vi "Send MC Telemetry.vi"   [LabVIEW 2014]
uses:
  MC Telemetry.ctl
  MC Temp 1.ctl
  MC Temp 2.ctl
  MC Temp 3.ctl
  MC Current.ctl
  MC Voltage.ctl
  MC State.ctl
  Inverter States.ctl
  Inverter Run Modes.ctl
  VSM States.ctl
  MC Torque.ctl
  MC Faults.ctl
  MC Post Faults.ctl
  MC Run Faults.ctl
  MC Position.ctl
  Global Data.vi
types:
  T1 = typedef "MC Telemetry.ctl" = cluster{"MC Temp 1":T2, "MC Temp 2":T3, "MC Temp 3":T4, "MC Current":T5, "MC Voltage":T6, "MC State":T7, "MC Torque":T11, "MC Faults":T12, "MC Position":T15}
  T2 = typedef "MC Temp 1.ctl" = cluster{"IGBT A (C)":dbl, "IGBT B (C)":dbl, "IGBT C (C)":dbl, "Gate Driver (C)":dbl}
  T3 = typedef "MC Temp 2.ctl" = cluster{"Control Board (C)":dbl, "RTD #1":dbl, "RTD #2":dbl, "RTD #3":dbl}
  T4 = typedef "MC Temp 3.ctl" = cluster{"RTD #4":dbl, "RTD #5":dbl, "Motor (C)":dbl, "T-Shudder":dbl}
  T5 = typedef "MC Current.ctl" = cluster{"I-Phase A":dbl, "I-Phase B":dbl, "I-Phase C":dbl, "I-Battery":dbl}
  T6 = typedef "MC Voltage.ctl" = cluster{"V-Phase AB":dbl, "V-Phase BC":dbl, "V-Output":dbl, "V-Battery":dbl}
  T7 = typedef "MC State.ctl" = cluster{"Inverter":T8, "Inv. Run Mode":T9, "Inv. Command":enum16{"CAN Mode", "VSM Mode"}, "Inv. Enable":enum16{"Inverter Disabled", "Inverter Enabled"}, "Inv. Enable Lock":enum16{"Inverter Locked", "Inverter Unlocked"}, "Direction":enum16{"Forward", "Reverse/Stopped"}, "VSM States":T10, "Relay 1":bool, "Relay 2":bool, "Relay 3":bool, "Relay 4":bool}
  T8 = typedef "Inverter States.ctl" = enum16{"Power On", "Stop", "Open Loop", "Closed Loop", "Wait", "Internal", "Idle Run", "Idle Stop", ""}
  T9 = typedef "Inverter Run Modes.ctl" = enum16{"Torque Mode", "Speed Mode"}
  T10 = typedef "VSM States.ctl" = enum16{"VSM Start", "Pre-Charge Init", "Pre-Charge Active", "Pre-Charge Complete", "VSM Wait", "VSM Ready", "Motor Running", "Blink Fault Code", "Shutdown in Process", "Recycle Power"}
  T11 = typedef "MC Torque.ctl" = cluster{"T-Requested (Telem)":dbl, "T-Feedback":dbl}
  T12 = typedef "MC Faults.ctl" = cluster{"POST":T13, "RUN":T14}
  T13 = typedef "MC Post Faults.ctl" = enum32{"None"}
  T14 = typedef "MC Run Faults.ctl" = enum32{"None"}
  T15 = typedef "MC Position.ctl" = cluster{"Motor Angle":dbl, "Motor Speed":dbl, "Electrical Output Freq.":dbl, "Delta Resolver Filt.":dbl}
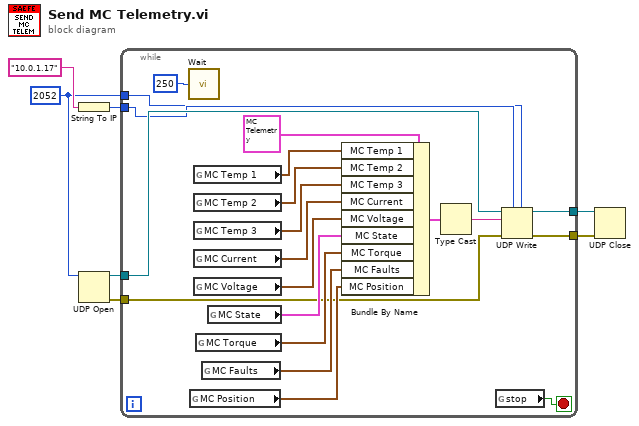
[diagram p0: block diagram]
diagram:
  w2 = u16 2052 ("port")
  n1 = String To IP(1:"10.0.1.17" ("name")) -> (0:w1:u32)
  n2 = UDP Open(11:w2) -> (port=w6:refnum<k16>, 0:w5:errorcluster)  [unwired: 4 in, 1 out]
  n3 = while {
    tunnel: w6 -> [w15]
    tunnel: w5 -> [w14]
    tunnel: [w11] -> w4
    tunnel: [w10] -> w3
    tunnel: w1 -> [w9]
    tunnel: w2 -> [w8]
    stop <- w26 stop-if-true
    n4 = call "Wait"("Count(mSec)"=u32 250) -> ()  [unwired: 1 out]
    n5 = global read "Global Data.vi" "MC Position"() -> (w16:T15)
    n6 = global read "Global Data.vi" "MC Temp 1"() -> (w24:T2)
    n7 = global read "Global Data.vi" "MC Temp 2"() -> (w23:T3)
    n8 = global read "Global Data.vi" "MC Temp 3"() -> (w22:T4)
    n9 = global read "Global Data.vi" "MC Current"() -> (w21:T5)
    n10 = global read "Global Data.vi" "MC Voltage"() -> (w20:T6)
    n11 = global read "Global Data.vi" "MC Torque"() -> (w18:T11)
    n12 = global read "Global Data.vi" "MC Faults"() -> (w17:T12)
    n13 = global read "Global Data.vi" "MC State"() -> (w19:T7)
    n14 = Bundle By Name(cluster=T1 {"MC Temp 1"={"IGBT A (C)"=0.0, "IGBT B (C)"=0.0, "IGBT C (C)"=0.0, "Gate Driver (C)"=0.0}, "MC Temp 2"={"Control Board (C)"=0.0, "RTD #1"=0.0, "RTD #2"=0.0, "RTD #3"=0.0}, "MC Temp 3"={"RTD #4"=0.0, "RTD #5"=0.0, "Motor (C)"=0.0, "T-Shudder"=0.0}, "MC Current"={"I-Phase A"=0.0, "I-Phase B"=0.0, "I-Phase C"=0.0, "I-Battery"=0.0}, "MC Voltage"={"V-Phase AB"=0.0, "V-Phase BC"=0.0, "V-Output"=0.0, "V-Battery"=0.0}, "MC State"={"Inverter"=enum."Power On", "Inv. Run Mode"=enum."Torque Mode", "Inv. Command"=enum."CAN Mode", "Inv. Enable"=enum."Inverter Disabled", "Inv. Enable Lock"=enum."Inverter Locked", "Direction"=enum."Forward", "VSM States"=enum."VSM Start", "Relay 1"=FALSE, "Relay 2"=FALSE, "Relay 3"=FALSE, "Relay 4"=FALSE}, "MC Torque"={"T-Requested (Telem)"=0.0, "T-Feedback"=0.0}, "MC Faults"={"POST"=enum."None", "RUN"=enum."None"}, "MC Position"={"Motor Angle"=0.0, "Motor Speed"=0.0, "Electrical Output Freq."=0.0, "Delta Resolver Filt."=0.0}} ("MC Telemetry"), "MC Temp 1"=w24, "MC Temp 2"=w23, "MC Temp 3"=w22, "MC Current"=w21, "MC Voltage"=w20, "MC State"=w19, "MC Torque"=w18, "MC Faults"=w17, "MC Position"=w16) -> (w13:T1)
    n15 = Type Cast(x=w13) -> (*(type *) &x=w12:string)  [unwired: 1 in]
    n16 = global read "Global Data.vi" "stop"() -> (w26:bool)
    n17 = UDP Write(address=w9, port or service name=w8, connection ID=w15, data in=w12, 8:w14) -> (error out=w10:errorcluster, 3:w11:refnum<k16>)  [unwired: 1 in]
  }
  n18 = UDP Close(connection ID=w4, 8:w3) -> ()  [unwired: 2 out]
